vi "simpletls test1.vi"() -> ()   [LabVIEW 2016]
uses:
  lvlibtls/client/lvlibretls client socket.lvclass
  C:/Users/IEUser/Desktop/tlssimple/libretls/context parent/lvlibretls configurable context.lvclass
  lvlibtls/socket connection/lvlibretls connection.lvclass
  lvlibtls/context parent/lvlibretls configurable context.lvclass
panel:
  out "error out":errorcluster
  out "data":string
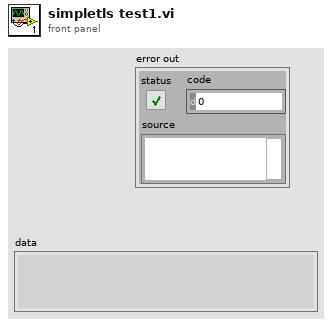
[diagram p1: front panel]
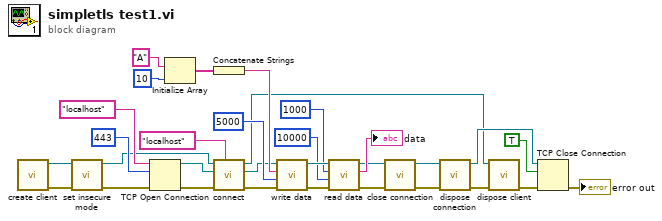
[diagram p0: block diagram]
diagram:
  n1 = call "create client.vi"() -> ("error out"=w9:errorcluster, "lvlibretls client socket out"=w2:refnum<class "lvlibretls client socket.lvclass">)  [unwired: 10 in]
  n2 = call "set insecure mode.vi"("error in"=w9, "lvlibretls configurable context in"=w2) -> ("error out"=w3:errorcluster, "lvlibretls configurable context out"=w1:refnum<class "lvlibretls client socket.lvclass">)  [unwired: 8 in]
  n3 = TCP Open Connection(address="localhost", remote port or service name=u16 443, error in (no error)=w3) -> (connection ID=w7:refnum<k5>, error out=w8:errorcluster)  [unwired: 2 in]
  n4 = Initialize Array("A" ("address"), 10 ("dimension size")) -> (w27:string[])
  n5 = Concatenate Strings(w27) -> (w20:string)
  n6 = call "connect.vi"("server name"="localhost", "error in"=w8, "connection ID"=w7, "lvlibretls client socket"=w1) -> ("error out"=w6:errorcluster, "lvlibretls connection"=w5:refnum<class "lvlibretls connection.lvclass">, "lvlibretls client socket out"=w4:refnum<class "lvlibretls client socket.lvclass">)  [unwired: 5 in]
  n7 = call "write data.vi"("error in"=w6, "timeout"=5000, "data"=w20, "lvlibretls connection in"=w5) -> ("error out"=w22:errorcluster, "lvlibretls connection out"=w25:refnum<class "lvlibretls connection.lvclass">)  [unwired: 6 in]
  n8 = call "read data.vi"("error in"=w22, "timeout"=10000, "max size"=1000, "lvlibretls connection in"=w25) -> ("error out"=w17:errorcluster, "data"=→"data":string, "lvlibretls connection out"=w18:refnum<class "lvlibretls connection.lvclass">)  [unwired: 5 in]
  n9 = call "close connection.vi"("error in"=w17, "lvlibretls connection in"=w18) -> ("error out"=w15:errorcluster, "lvlibretls connection out"=w16:refnum<class "lvlibretls connection.lvclass">)  [unwired: 8 in]
  n10 = call "dispose connection.vi"("error in"=w15, "lvlibretls connection in"=w16) -> ("error out"=w12:errorcluster, "connection"=w14:refnum<k5>)  [unwired: 8 in]
  n11 = call "dispose client.vi"("error in"=w12, "lvlibretls client socket in"=w4) -> ("error out"=w11:errorcluster)  [unwired: 9 in]
  n12 = TCP Close Connection(connection ID=w14, abort (F)=TRUE, error in (no error)=w11) -> (error out=→"error out":errorcluster)  [unwired: 1 out]
